vi "Send XY Position Command.vi"(8 "error in (no error)":errorcluster, 9 "Polarization":u16(ring) items=["Vertical", "Horizontal"], 10 "Position":i32=1 caption="Antenna\nPosition 1 - 16" min=0 max=16 step=1, 11 "MotionComm in":refnum<class "MotionComm.lvclass">) -> (0 "error out":errorcluster, 3 "MotionComm out":refnum<class "MotionComm.lvclass">)   [LabVIEW 2017]
doc: "Send a command to the VXM thread,\nthen wait for an ack back on the VXM Ack que"
uses:
  Support/MessageQue/MessageQue.lvlib
  MotionComm.lvclass
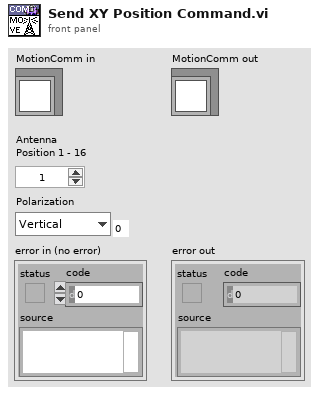
[diagram p1: front panel]
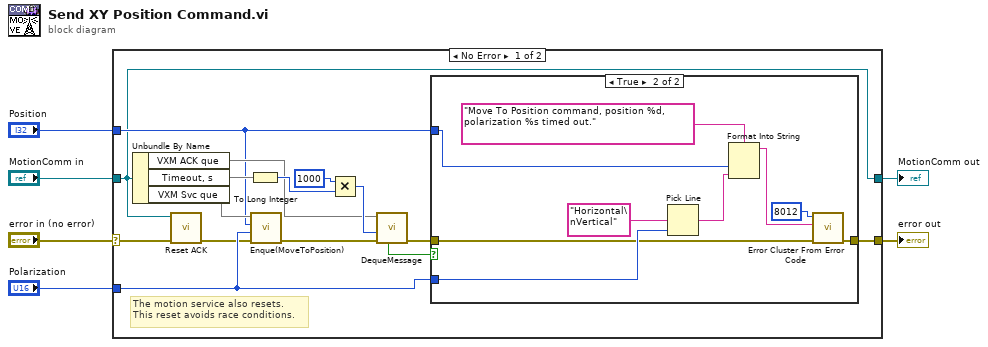
[diagram p0: block diagram]
diagram:
  n1 = case shown="No Error" "error in (no error)" {
    selector: "error in (no error)" -> [w8 w33]
    tunnel: [w10 w33] -> w5
    tunnel: [w7 w32] -> w3
    tunnel: "MotionComm in" -> [w7 w32]
    tunnel: "Position" -> [w13 _]
    tunnel: "Polarization" -> [w14 _]
    frame No Error {
      # "The motion service also resets.\nThis reset avoids race conditions."
      n2 = Unbundle By Name(w7) -> ("VXM ACK que"=w15, "Timeout, s"=w16, "VXM Svc que"=w21)
      n3 = call "Reset ACK.vi"("error in (no error)"=w8, "MotionComm in"=w7) -> ("error out"=w9:errorcluster)  [unwired: 8 in, 1 out]
      n4 = To Long Integer(number=w16) -> (32bit integer=w18:i32)
      n5 = call "Enque(MoveToPosition).vi"("error in"=w9, "Polarization"=w14, "Position"=w13, "Message que"=w21) -> ("error out"=w20:errorcluster)  [unwired: 6 in, 1 out]
      n6 = Multiply(x=1000 ("timeout in ms (-1)"), y=w18) -> (x*y=w17:i32)
      n7 = call "DequeMessage.vi"("error in"=w20, "timeout in ms (-1)"=w17, "Message que"=w15) -> ("error out"=w11:errorcluster, "timed out?"=w12:bool)  [unwired: 3 in, 4 out]
      n8 = case shown="True" w12 {
        tunnel: w14 -> [_ w28]
        tunnel: w13 -> [_ w27]
        tunnel: w11 -> [w22 w24]
        tunnel: [w22 w23] -> w10
        frame False {
        }
        frame True {
          n9 = Pick Line(multi-line string="Horizontal\nVertical" ("format string"), line index=w28) -> (output string=w26:string)  [unwired: 1 in]
          n10 = Format Into String(format string="Move To Position command, position %d, polarization %s timed out.", w27, w26) -> (resulting string=w25:string)  [unwired: 2 in, 1 out]
          n11 = call <vilib>:"Error Cluster From Error Code.vi"("error in (no error)"=w24, "error message (\"\")"=w25, "error code (0)"=8012) -> ("error out"=w23:errorcluster)  [unwired: 6 in]
        }
      }
    }
    frame Error {
    }
  }
  "error out" <- w5
  "MotionComm out" <- w3
